vi "Revision Query.vi"(8 "error in (no error)":errorcluster, 11 "VISA resource name":refnum<visa-resource-name>) -> (0 "error out":errorcluster, 1 "Instr Firmware Revision":string, 2 "Instr Driver Revision":string, 3 "VISA resource name out":refnum<visa-resource-name>, 4 "Instr Serial Number":string, 5 "Instr Option":string, 6 "FPGA Firmware Revision":string, 7 "Instr Model":string)   [LabVIEW 2012, in "Quantum Composers 9000 Series.lvlib"]
doc: "This VI queries the current instrument firmware revision and instrument driver revision.\n\nThis Instrument Driver's Revision number is 1.0 and is compatible with Instrument Firmware Revision 1.20\n\nDriver Name: Quantum Composers 9000 Series\nCreated By: RME\nRelease Date: 4/06\nOriginally Developed in LabVIEW Version: 8.0\n\nModification History:"
uses:
  <instrlib>/Quantum Composers 9000 Series/Quantum Composers 9000 Series.lvlib
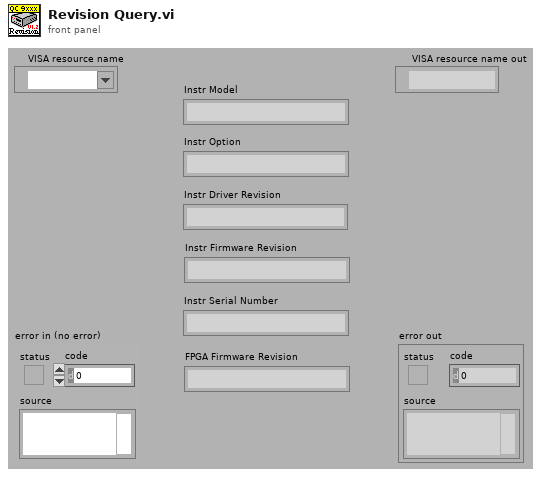
[diagram p1: front panel]
types:
  T1 = cluster{"Major":u16, "Minor":u16, "Fix":u16, "Build":u16}
  T2 = typedef "Quantum Composers 9000 Series.lvlib/Unit Info.ctl" = cluster{"ID String":string, "Model":string, "Model #":i32, "# Channels":i32, "Options":string, "Firmware":string, "FPGA Ver":string}
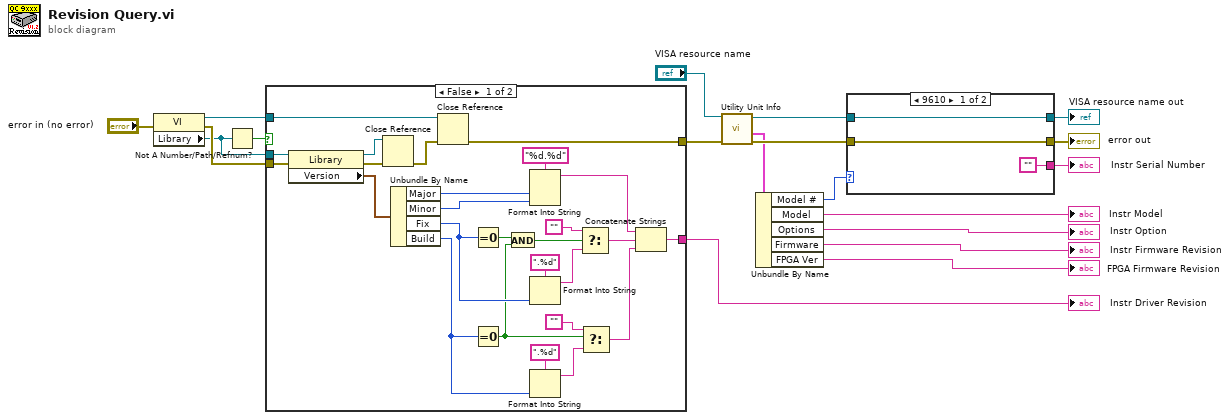
[diagram p0: block diagram]
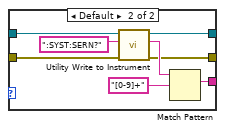
[diagram p2: hidden frame]
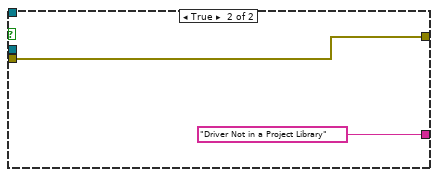
[diagram p3: hidden frame]
diagram:
  n1 = property on="Property Node" class="VI"(error in="error in (no error)") -> (reference out=w19:refnum<vi>, error out=w18:errorcluster, "Library"=w17:refnum<vi>)  [unwired: 1 in]
  n2 = Not A Number/Path/Refnum?(number/path/refnum=w17) -> (NaN/Path/Refnum?=w16:bool)
  n3 = case shown="False" w16 {
    tunnel: w19 -> [w42 _]
    tunnel: w18 -> [w27 w47]
    tunnel: [w22 w47] -> w13
    tunnel: [w21 "Driver Not in a Project Library"] -> w15
    tunnel: w17 -> [w20 _]
    frame False {
      n4 = property on="Property Node" class="Library"(reference=w20, error in=w27) -> (reference out=w44:refnum<vi>, error out=w45:errorcluster, "Version"=w41:T1)
      n5 = Close Reference(reference=w44, error in (no error)=w45) -> (error out=w43:errorcluster)
      n6 = Unbundle By Name(w41) -> ("Major"=w30:u16, "Minor"=w29:u16, "Fix"=w26:u16, "Build"=w28:u16)
      n7 = Close Reference(reference=w42, error in (no error)=w43) -> (error out=w22:errorcluster)
      n8 = Equal To 0?(x=w26) -> (x = 0?=w25:bool)
      n9 = Equal To 0?(x=w28) -> (x = 0?=w24:bool)
      n10 = And(x=w25, y=w24) -> (x .and. y?=w23:bool)
      n11 = Format Into String(format string="%d.%d", w30, w29) -> (resulting string=w36:string)  [unwired: 2 in, 1 out]
      n12 = Format Into String(format string=".%d", w26) -> (resulting string=w38:string)  [unwired: 2 in, 1 out]
      n13 = Format Into String(format string=".%d", w28) -> (resulting string=w34:string)  [unwired: 2 in, 1 out]
      n14 = Select(t="", s=w23, f=w38) -> (s? t:f=w35:string)
      n15 = Select(t="", s=w24, f=w34) -> (s? t:f=w31:string)
      n16 = Concatenate Strings(w36, w35, w31) -> (w21:string)
    }
    frame True {
    }
  }
  "Instr Driver Revision" <- w15
  n17 = call <instrlib>:"Utility Unit Info.vi"("Error In (no error)"=w13, "VISA resource name in"="VISA resource name") -> ("Error Out"=w12:errorcluster, "Unit Info Out"=w10:T2, "VISA resource name out"=w7:refnum<visa-resource-name>)  [unwired: 7 in]
  n18 = Unbundle By Name(w10) -> ("Model #"=w1:i32, "Model"=→"Instr Model":string, "Options"=→"Instr Option":string, "Firmware"=→"Instr Firmware Revision":string, "FPGA Ver"=→"FPGA Firmware Revision":string)
  n19 = case shown="9610" w1 {
    tunnel: w12 -> [w49 w55]
    tunnel: [w49 w54] -> w9
    tunnel: [w50 w53] -> w8
    tunnel: w7 -> [w50 w52]
    tunnel: ["" w51] -> w6
    frame 9610 {
    }
    frame Default {
      n20 = call <instrlib>:"Utility Write to Instrument.vi"("error in (no error)"=w55, "Write Buffer"=":SYST:SERN?" ("Revision Query Command"), "VISA resource name"=w52) -> ("error out"=w54:errorcluster, "Read Buffer"=w56:string, "VISA resource name out"=w53:refnum<visa-resource-name>)  [unwired: 6 in]
      n21 = Match Pattern(string=w56, regular expression="[0-9]+") -> (match substring=w51:string)  [unwired: 1 in, 3 out]
    }
  }
  "VISA resource name out" <- w8
  "error out" <- w9
  "Instr Serial Number" <- w6
